vi "Get Double Data.vi"(8 "error in (no error)":errorcluster, 10 "Name":string, 11 "DoubleDictionary in":refnum<class "DoubleDictionary.lvclass">) -> (0 "error out":errorcluster, 2 "Value":dbl, 3 "DoubleDictionary out":refnum<class "DoubleDictionary.lvclass">)   [LabVIEW 2014, in "bmlv.lvlib" / "DoubleDictionary.lvclass"]
uses:
  DoubleDictionary.lvclass
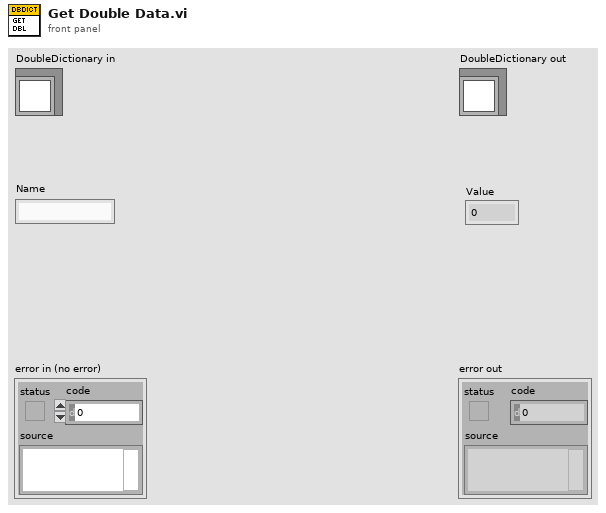
[diagram p1: front panel]
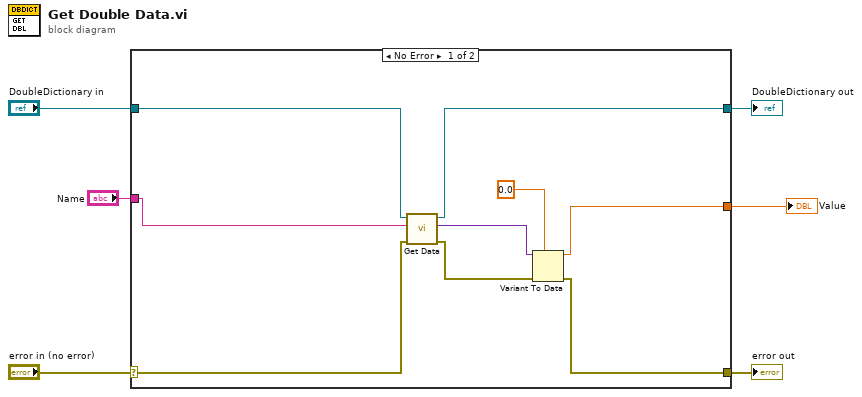
[diagram p0: block diagram]
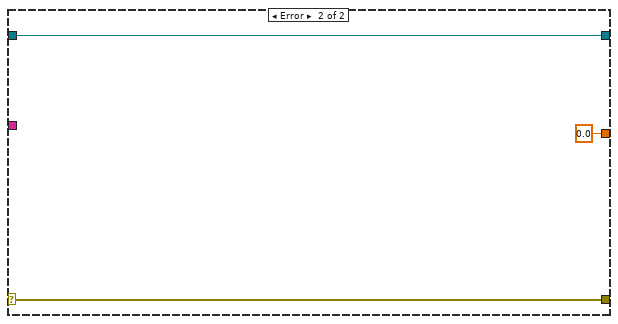
[diagram p2: hidden frame]
diagram:
  n1 = case shown="No Error" "error in (no error)" {
    selector: "error in (no error)" -> [w9 w18]
    tunnel: [w8 w18] -> w5
    tunnel: [w14 w17] -> w3
    tunnel: "DoubleDictionary in" -> [w15 w17]
    tunnel: "Name" -> [w13 _]
    tunnel: [w7 0.0] -> w1
    frame No Error {
      n2 = call-dynamic "Get Data.vi"("error in (no error)"=w9, "Name"=w13, "Dictionary in"=w15) -> ("error out"=w10:errorcluster, "Value"=w11:variant, "Dictionary out"=w14:refnum<class "DoubleDictionary.lvclass">)  [unwired: 6 in]
      n3 = Variant To Data(error in=w10, type=0.0, Variant=w11) -> (data=w7:dbl, error out=w8:errorcluster)
    }
    frame Error {
    }
  }
  "error out" <- w5
  "DoubleDictionary out" <- w3
  "Value" <- w1
